vi "test Source Separated.vi"(8 "error in (no error)":errorcluster, 11 "TestCase in":refnum<class "Code Compliance Test Case.lvclass">) -> (0 "error out":errorcluster, 3 "TestCase out":refnum<class "Code Compliance Test Case.lvclass">)   [LabVIEW 2027, in "Code Compliance Test Case.lvclass"]
uses:
  Code Compliance Test Case.lvclass
  C:/Program Files/National Instruments/LabVIEW 2027/vi.lib/addons/_JKI Toolkits/VI Tester/TestCase.llb/TestCase.lvclass
  <vilib>/addons/_JKI Toolkits/VI Tester/TestCase.llb/TestCase.lvclass
  <vilib>/NI/VeriStand Custom Device Testing Tools/VeriStandTestUtilities/VeriStandTestUtilities.lvlib
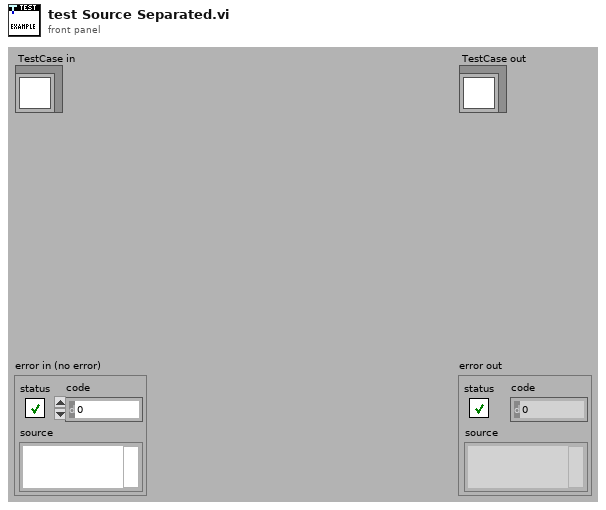
[diagram p1: front panel]
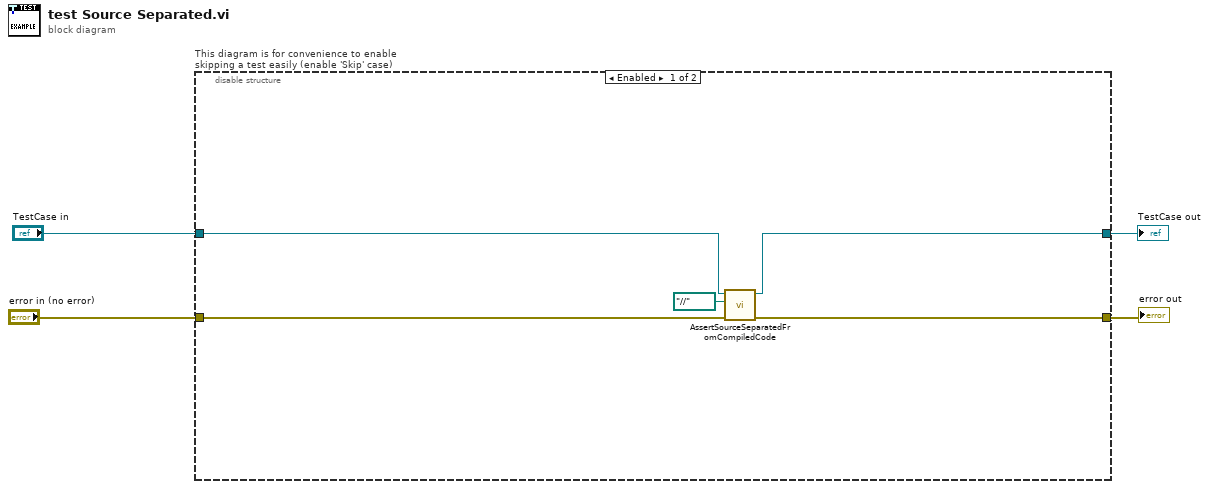
[diagram p0: block diagram]
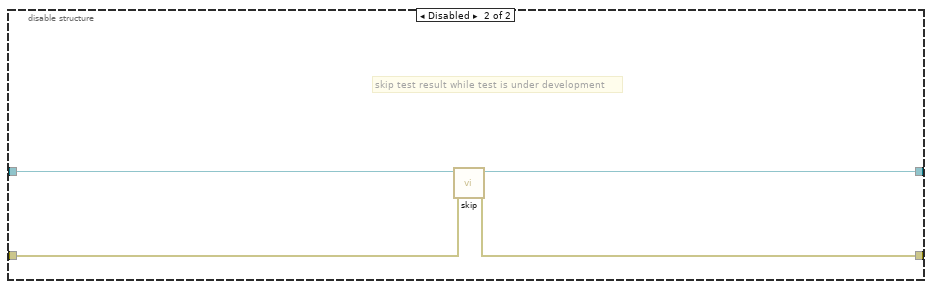
[diagram p2: hidden frame]
diagram:
  n1 = disable-structure "This diagram is for convenience to enable skipping a test easily (enable 'Skip' case)" shown="Enabled" {
    disable-tunnel: "TestCase in" -> [w7 w13]
    disable-tunnel: [w5 w11] -> w1
    disable-tunnel: [w6 w12] -> w3
    disable-tunnel: "error in (no error)" -> [w8 w10]
    frame Enabled {
      n2 = call <vilib>:"AssertSourceSeparatedFromCompiledCode.vi"("error in"=w8, "search path"=path "../../..", "TestCase in"=w7) -> ("error out"=w6:errorcluster, "TestCase out"=w5:refnum<class "Code Compliance Test Case.lvclass">)  [unwired: 7 in]
    }
    frame Disabled {
      # "skip test result while test is under development"
      n3 = call <vilib>:"skip.vi"("error in (no error)"=w10, "TestCase in"=w13) -> ("error out"=w12:errorcluster, "TestCase out"=w11:refnum<class "Code Compliance Test Case.lvclass">)  [unwired: 8 in]
    }
  }
  "error out" <- w3
  "TestCase out" <- w1
